vi "Is equal.vi"(4 "address 2":refnum<class "Generic Network Address.lvclass">, 5 "address":refnum<class "MacOS Network Address.lvclass">) -> (1 "equal?":bool)   [LabVIEW 2020, in "NI_WFCN.lvlib" / "MacOS Network Address.lvclass"]
doc: "Returns TRUE if the addresses are equal."
uses:
  <vilib>/net/WFCN/Addressing/MacOS Network Address/MacOS Network Address.lvclass
  <vilib>/net/WFCN/Addressing/Generic Network Address/Generic Network Address.lvclass
  <vilib>/net/WFCN/Addressing/MacOS Network Address/MacOS Network Address.lvclass/MacOS Network Address.ctl
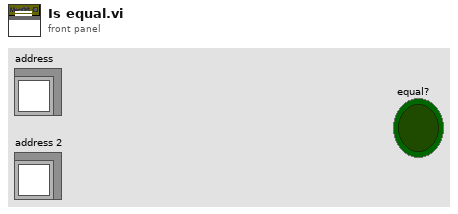
[diagram p1: front panel]
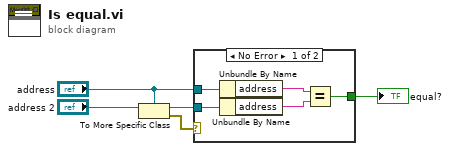
[diagram p0: block diagram]
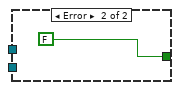
[diagram p2: hidden frame]
diagram:
  n1 = To More Specific Class(target class="address", reference="address 2") -> (specific class reference=w4:refnum<class "MacOS Network Address.lvclass">, error out=w5:errorcluster)  [unwired: 1 in]
  n2 = case shown="No Error" w5 {
    tunnel: w4 -> [w9 _]
    tunnel: "address" -> [w10 _]
    tunnel: [w6 FALSE] -> w1
    frame No Error {
      n3 = Unbundle By Name(w10) -> ("address"=w8:string)
      n4 = Unbundle By Name(w9) -> ("address"=w7:string)
      n5 = Equal?(x=w8, y=w7) -> (x = y?=w6:bool)
    }
    frame Error {
    }
  }
  "equal?" <- w1
